vi "PAN_FindCmdSet2.vi"(10 "cmdset":string="single_tcp") -> (0 "error resp out":errorcluster, 1 "error cmd out":errorcluster, 2 "respref":refnum<vi>, 3 "cmdref":refnum<vi>, 5 "async reference":refnum<vi>, 7 "error async out":errorcluster)   [LabVIEW 2016]
panel:
  in  "type specifier VI Refnum (for type only) 3":refnum<vi>
  in  "type specifier VI Refnum (for type only) 2":refnum<vi>
  in  "type specifier VI Refnum (for type only)":refnum<vi>
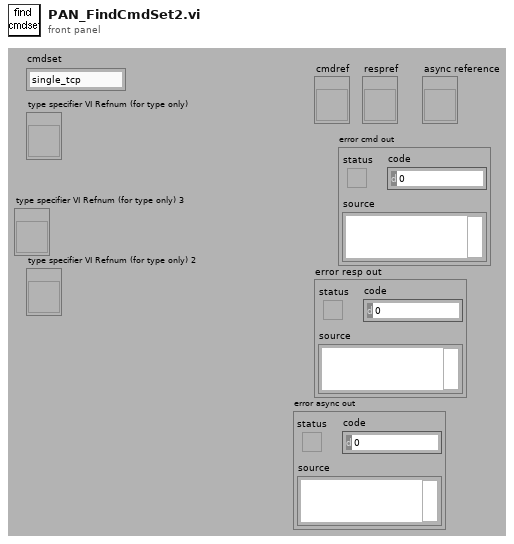
[diagram p1: front panel]
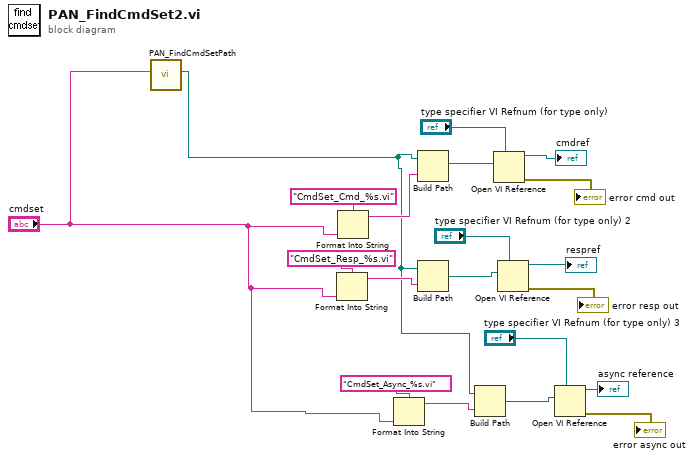
[diagram p0: block diagram]
diagram:
  n1 = call "PAN_FindCmdSetPath.vi"("cmdset name"="cmdset") -> ("path"=w1:path)  [unwired: 10 out]
  n2 = Format Into String(format string="CmdSet_Resp_%s.vi", "cmdset") -> (resulting string=w17:string)  [unwired: 2 in, 1 out]
  n3 = Format Into String(format string="CmdSet_Cmd_%s.vi", "cmdset") -> (resulting string=w18:string)  [unwired: 2 in, 1 out]
  n4 = Format Into String(format string="CmdSet_Async_%s.vi", "cmdset") -> (resulting string=w9:string)  [unwired: 2 in, 1 out]
  n5 = Build Path(base path=w1, name or relative path=w18) -> (appended path=w16:path)
  n6 = Build Path(base path=w1, name or relative path=w17) -> (appended path=w15:path)
  n7 = Build Path(base path=w1, name or relative path=w9) -> (appended path=w8:path)
  n8 = Open VI Reference(type specifier VI Refnum (for type only)="type specifier VI Refnum (for type only)", vi path=w16) -> (vi reference=→"cmdref":refnum<vi>, error out=→"error cmd out":errorcluster)  [unwired: 1 in, 3 out]
  n9 = Open VI Reference(type specifier VI Refnum (for type only)="type specifier VI Refnum (for type only) 2", vi path=w15) -> (vi reference=→"respref":refnum<vi>, error out=→"error resp out":errorcluster)  [unwired: 1 in, 3 out]
  n10 = Open VI Reference(type specifier VI Refnum (for type only)="type specifier VI Refnum (for type only) 3", vi path=w8) -> (vi reference=→"async reference":refnum<vi>, error out=→"error async out":errorcluster)  [unwired: 2 in, 2 out]
